vi "max_array_size.vi"(9 "max rows":u32=8, 10 "Array":string[](array[string])) -> (1 "size > max rows":bool, 2 "array size":u32)   [LabVIEW 2015]
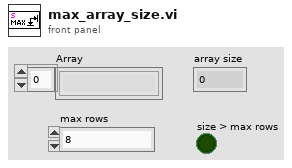
[diagram p1: front panel]
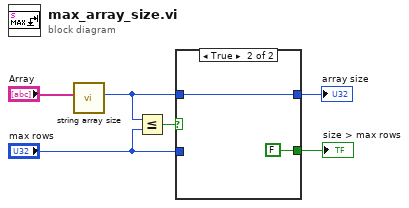
[diagram p0: block diagram]
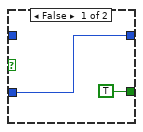
[diagram p2: hidden frame]
diagram:
  n1 = call "string array size.vi"("array"="Array") -> ("size"=w1:u32)  [unwired: 10 in]
  n2 = Less Or Equal?(x=w1, y="max rows") -> (x <= y?=w6:bool)
  n3 = case shown="True" w6 {
    tunnel: w1 -> [_ w10]
    tunnel: [w7 w10] -> w5
    tunnel: [TRUE FALSE] -> w4
    tunnel: "max rows" -> [w7 _]
    frame False {
    }
    frame True {
    }
  }
  "array size" <- w5
  "size > max rows" <- w4
